vi "Read rec0MQ.vi"(8 "error in (no error)":errorcluster, 11 "Messenger in":refnum<class "Messenger.lvclass">) -> (0 "error out":errorcluster, 2 "rec0MQ":bool, 3 "Messenger out":refnum<class "Messenger.lvclass">)   [LabVIEW 2018, in "Messenger.lvclass"]
uses:
  Messenger.lvclass
  Messenger.lvclass/Messenger.ctl
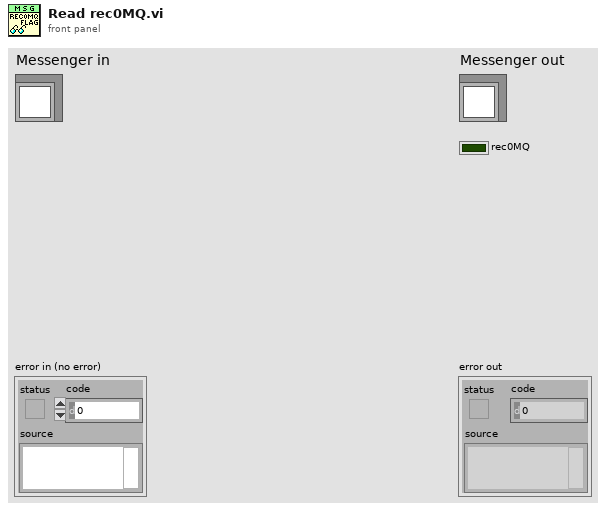
[diagram p1: front panel]
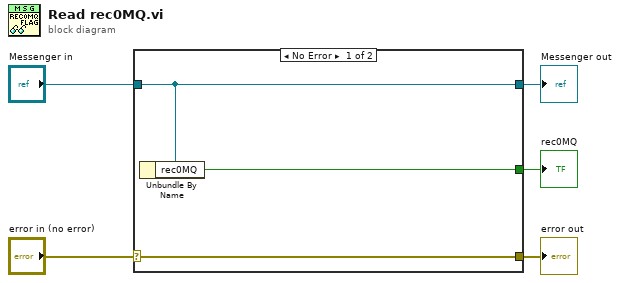
[diagram p0: block diagram]
diagram:
  n1 = case shown="No Error" "error in (no error)" {
    selector: "error in (no error)" -> [w8 w9]
    tunnel: [w8 w9] -> w4
    tunnel: [w7 w10] -> w2
    tunnel: "Messenger in" -> [w7 w10]
    tunnel: [w6 _] -> w1
    frame No Error {
      n2 = Unbundle By Name(w7) -> ("rec0MQ"=w6:bool)
    }
    frame Error {
    }
  }
  "error out" <- w4
  "Messenger out" <- w2
  "rec0MQ" <- w1
